vi "TUNA midbrain SENSE.vi"(0 "Boat Status":T1={"GPS"={"X pos"=0, "Y pos"=0, "Heading"=0.0}, "IR Sensors"=[{"Name"="Bow", "Angle"=0.0, "Distance"=0.0}], "MOT BAT"=7.2, "RIO BAT"=7.2}, 1 "error in":errorcluster) -> (2 "IR Sensors":T2(array[cluster]), 3 "Battery\nDead?":bool, 4 "error out":errorcluster)   [LabVIEW 2014]
doc: "This VI receives the status of the boat from the Hindbrain and determines:\n1. Is the boat stuck?\n2. Is the battery dead?"
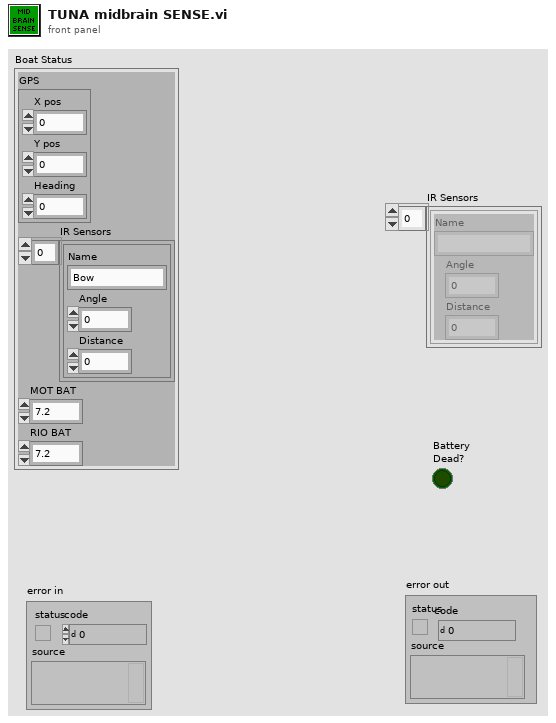
[diagram p1: front panel]
types:
  T1 = cluster{"GPS":cluster{"X pos":i32, "Y pos":i32, "Heading":dbl}, "IR Sensors":cluster{"Name":string, "Angle":dbl, "Distance":dbl}[], "MOT BAT":dbl, "RIO BAT":dbl}
  T2 = cluster{"Name":string, "Angle":dbl, "Distance":dbl}[]
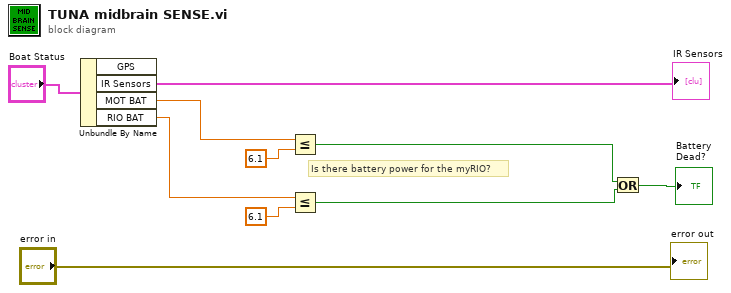
[diagram p0: block diagram]
diagram:
  # "Is there battery power for the myRIO?"
  n1 = Unbundle By Name("Boat Status") -> ("IR Sensors"=→"IR Sensors":T2, "MOT BAT"=w8:dbl, "RIO BAT"=w4:dbl)  [unwired: 1 out]
  n2 = Less Or Equal?(x=w8, y=6.1) -> (x <= y?=w3:bool)
  n3 = Less Or Equal?(x=w4, y=6.1) -> (x <= y?=w2:bool)
  n4 = Or(x=w3, y=w2) -> (x .or. y?=→"Battery\nDead?":bool)
  "error out" <- "error in"
